vi "Wait for Result.vi"(11 "Async Authorization in":refnum<class "Async Authorization.lvclass">) -> (0 "error out":errorcluster, 2 "Authorization":refnum<class "Authorization.lvclass">, 3 "Async Authorization out":refnum<class "Async Authorization.lvclass">)   [LabVIEW 2020, in "OAuth2.lvlib" / "Async Authorization.lvclass"]
uses:
  Async Authorization.lvclass
  Async Authorization.lvclass/Async Authorization.ctl
  Authorization/Authorization.lvclass
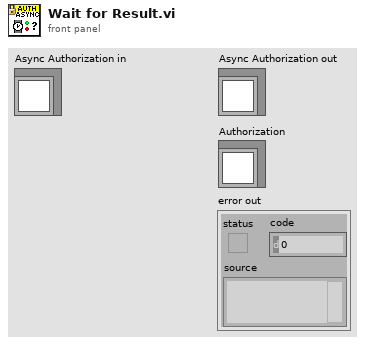
[diagram p1: front panel]
types:
  T1 = typedef "OAuth2.lvlib/Async Auth Result.ctl" = cluster{"Authorization":refnum<class "Authorization.lvclass">, "error":errorcluster}
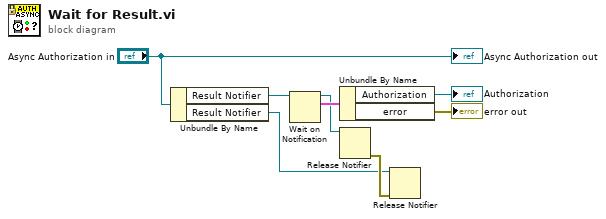
[diagram p0: block diagram]
diagram:
  n1 = Unbundle By Name("Async Authorization in") -> ("Result Notifier"=w7:refnum<notifier>, "Result Notifier"=w1:refnum<notifier>)
  n2 = Wait on Notification(notifier=w7) -> (notifier out=w3:refnum<notifier>, notification=w6:T1)  [unwired: 3 in, 2 out]
  n3 = Unbundle By Name(w6) -> ("Authorization"=→"Authorization":refnum<class "Authorization.lvclass">, "error"=→"error out":errorcluster)
  n4 = Release Notifier(notifier=w3) -> (error out=w2:errorcluster)  [unwired: 2 in, 2 out]
  n5 = Release Notifier(notifier=w1, error in (no error)=w2) -> ()  [unwired: 1 in, 3 out]
  "Async Authorization out" <- "Async Authorization in"
